vi "PIV_close.vi"(8 "error in (no error)":errorcluster) -> (0 "error out":errorcluster, 3 "reply":string)   [LabVIEW 2025]
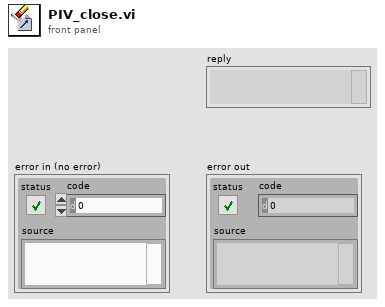
[diagram p1: front panel]
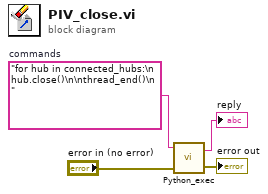
[diagram p0: block diagram]
diagram:
  w1 = "for hub in connected_hubs:\n    hub.close()\n\nthread_end()\n    "  # commands
  n1 = call "Python_exec.vi"("error in (no error)"="error in (no error)", "commands"=w1) -> ("error out"=→"error out":errorcluster, "reply"=→"reply":string)  [unwired: 1 in]
